vi "DDE Close Conversation.vi"(6 "error in (no error)":errorcluster, 8 "mode(T,close immediately)":bool=TRUE, 9 "conversation refnum":u32) -> (0 "error out":errorcluster)   [LabVIEW 2014]
doc: "Closes a DDE conversation. Refer to the Using DDE in LabVIEW Application Note for more information about DDE.\n\n<B>conversation refnum</B> is a refnum that uniquely identifies this DDE conversation.\n\nIf <B>mode</B> is TRUE (default), the DDE conversation always is closed. If FALSE, the conversation closes only when an error passes in. Therefore, if you wire the <B>error out</B> of another DDE VI to the <B>error in</B> of this VI with a FALSE <B>mode</B>, the conversation terminates only if an error occurs in the first VI.\n\n<B>error in</B> describes error conditions that occur before this VI or function runs. The default is no error. If an error occurred before this VI or function runs, the VI or function passes the <B>error in</B> value to <B>error out</B>. This VI or function runs normally only if no error occurs before this VI or function runs. If an error occurs while this VI or function runs, it runs normally and sets its own error status in <B>error out</B>. Use the Simple Error Handler or General Error Handler VIs to display the description of the error code. Use <B>error in</B> and <B>error out</B> to check errors and to specify execution order by wiring <B>error out</B> from one node to <B>error in</B> of the next node.\n\n<B>status</B> is TRUE (X) if an error occurred before this VI or function ran or FALSE (checkmark) to indicate a warning or that no error occurred before this VI or function ran. The default is FALSE.\n\n<B>code</B> is the error or warning code. The default is 0. If <B>status</B> is TRUE, <B>code</B> is a non-zero error code. If <B>status</B> is FALSE, <B>code</B> is 0 or a warning code.\n\n<B>source</B> describes the origin of the error or warning and is, in most cases, the name of the VI or function that produced the error or warning. The default is an empty string.\n\n<B>error out</B> contains error information. If <B>error in</B> indicates that an error occurred before this VI or function ran, <B>error out</B> contains the same error information. Otherwise, it describes the error status that this VI or function produces. Right-click the <B>error out</B> indicator on the front panel and select <B>Explain Error</B> from the shortcut menu for more information about the error.\n\n<B>status</B> is TRUE (X) if an error occurred or FALSE (checkmark) to indicate a warning or that no error occurred.\n\n<B>code</B> is the error or warning code. If <B>status</B> is TRUE, <B>code</B> is a non-zero error code. If <B>status</B> is FALSE, <B>code</B> is 0 or a warning code.\n\n<B>source</B> describes the origin of the error or warning and is, in most cases, the name of the VI or function that produced the error or warning."
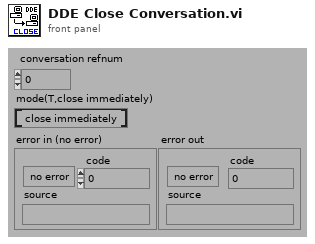
[diagram p1: front panel]
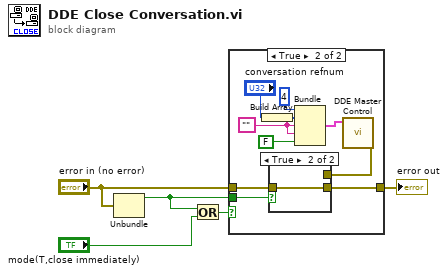
[diagram p0: block diagram]
diagram:
  n1 = Unbundle("error in (no error)") -> ("status"=w1:bool)  [unwired: 2 out]
  n2 = Or(x=w1, y="mode(T,close immediately)") -> (x .or. y?=w3:bool)
  n3 = case shown="True" w3 {
    tunnel: [w6 w10] -> w4
    tunnel: "error in (no error)" -> [w6 w11]
    tunnel: w1 -> [_ w12]
    frame False {
    }
    frame True {
      w14 = ""
      n4 = Build Array("conversation refnum") -> (w7:u32[])
      n5 = Bundle(i8 4, w7, w14, w14, FALSE) -> (w16:cluster{i8, u32[], string, string, bool})  [unwired: 1 in]
      n6 = call "DDE Master Control.vi"("input"=w16) -> ("error out"=w9:errorcluster)  [unwired: 4 in, 4 out]
      n7 = case shown="True" w12 {
        tunnel: w11 -> [_ w18]
        tunnel: [w17 w18] -> w10
        tunnel: w9 -> [w17 _]
        frame False {
        }
        frame True {
        }
      }
    }
  }
  "error out" <- w4
